vi "VMI_find_peaks.vi"(2 "Acquire Time":i32, 3 "Acquire Queue In":T2, 4 "Peak Find Settings":T1, 6 "Image Queue in":T2, 7 "Peak Position Queue in":T2) -> (0 "error out":errorcluster, 1 "x-y":u32)   [LabVIEW 2020]
uses:
  <vilib>/vision/Image Controls.llb/IMAQ Image.ctl
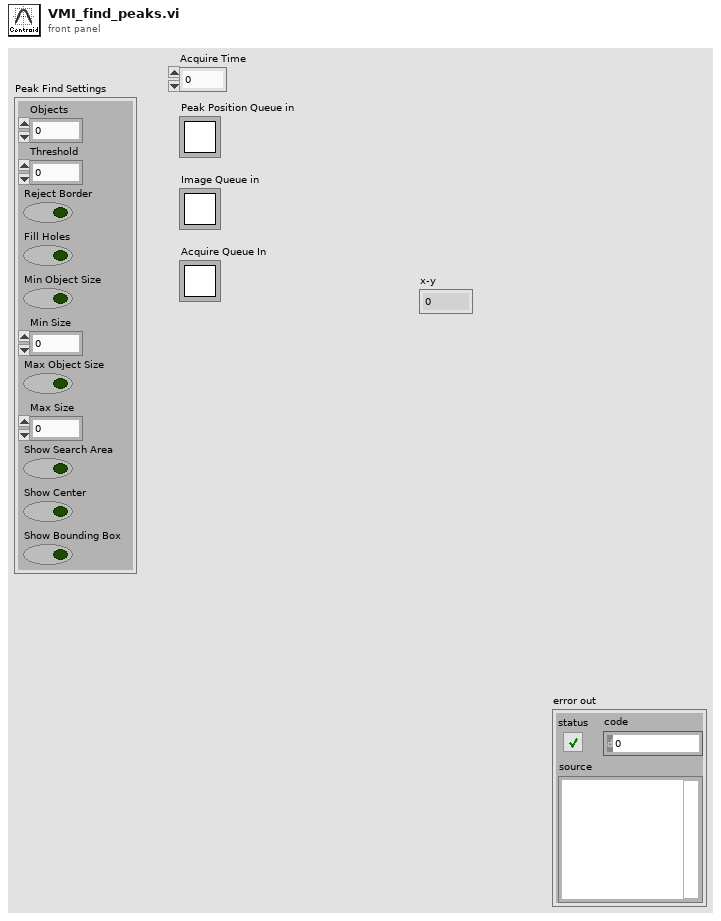
[diagram p1: front panel]
types:
  T1 = cluster{"Objects":u16, "Threshold":i32, "Reject Border":bool, "Fill Holes":bool, "Min Object Size":bool, "Min Size":i32, "Max Object Size":bool, "Max Size":i32, "Show Search Area":bool, "Show Center":bool, "Show Bounding Box":bool}
  T2 = typedef "Queue RefNum" = refnum<k1>
  T3 = typedef "IMAQ Image.ctl" = refnum<image>
  T4 = cluster{"Object Center":cluster{"X":sgl, "Y":sgl}, "Bounding Box":cluster{"X Left":i32, "Y Top":i32, "X Right":i32, "Y Bottom":i32}, "Area":sgl, "Orientation":sgl, "Aspect Ratio":sgl, "Nb Holes":i32}[]
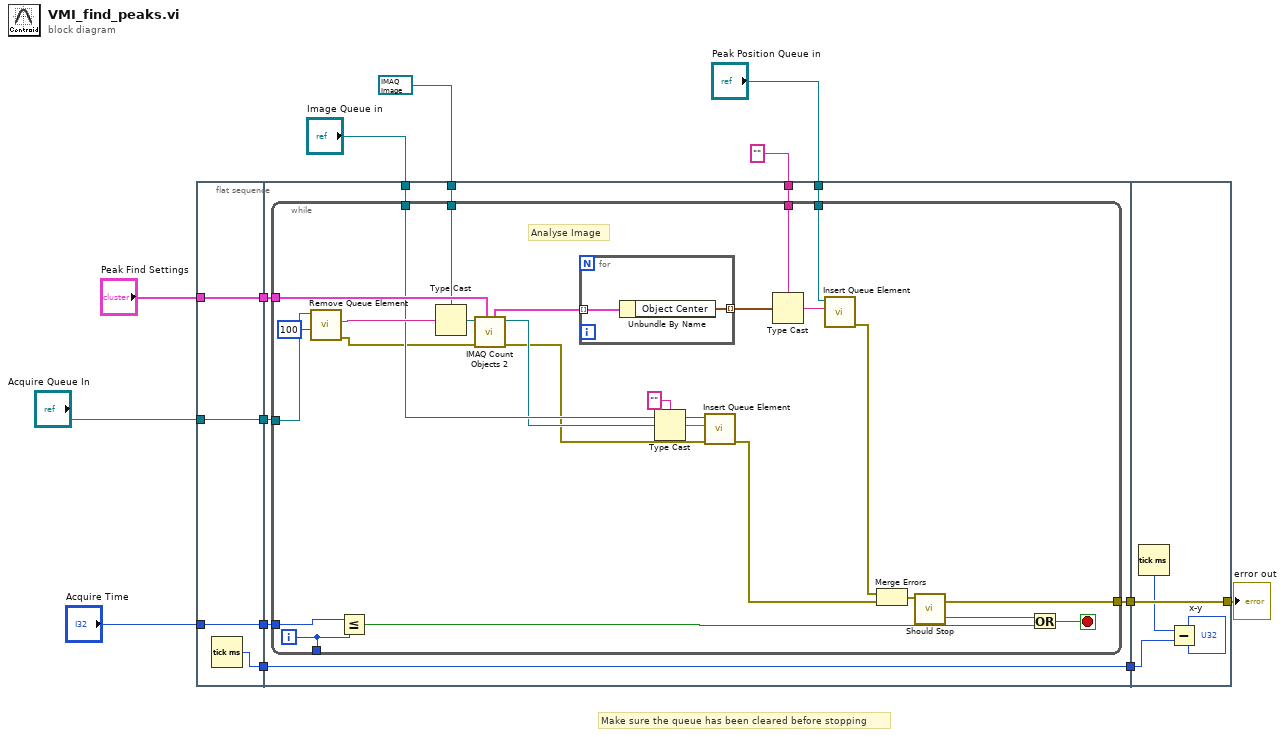
[diagram p0: block diagram]
diagram:
  # "Make sure the queue has been cleared before stopping"
  n1 = flat-sequence {
    tunnel: "Acquire Time" -> [w16]
    tunnel: "Peak Find Settings" -> [w17]
    tunnel: "Acquire Queue In" -> [w18]
    tunnel: [w18] -> w7
    tunnel: [w17] -> w6
    tunnel: [w16] -> w5
    tunnel: [w15] -> w3
    tunnel: "Image Queue in" -> [w27]
    tunnel: "Peak Position Queue in" -> [w23]
    tunnel: [w25] -> w8
    tunnel: w7 -> [w26]
    tunnel: w6 -> [w24]
    tunnel: w5 -> [w22]
    tunnel: [w21] -> w4
    tunnel: w3 -> [w21]
    tunnel: T3 refnum ("Image Out") -> [w20]
    tunnel: "" -> [w19]
    tunnel: [w59] -> w12
    tunnel: w8 -> [w59]
    tunnel: w4 -> [w57]
    frame #0 {
      n2 = Tick Count (ms)() -> (millisecond timer value=w15:u32)
    }
    frame #1 {
      n3 = while {
        tunnel: w26 -> [w40]
        tunnel: w24 -> [w51]
        tunnel: w23 -> [w48]
        tunnel: w27 -> [w46]
        tunnel: [w34] -> w25
        tunnel: w22 -> [w37]
        tunnel: [w33] -> _
        tunnel: w20 -> [w30]
        tunnel: w19 -> [w29]
        i -> [w33]
        stop <- w38 stop-if-true
        # "Analyse Image"
        n4 = call <vilib>:"Remove Queue Element.vi"("ms timeout (-1)"=100, "queue"=w40) -> ("error out"=w44:errorcluster, "queue element"=w53:string)  [unwired: 4 in, 2 out]
        n5 = Less Or Equal?(x=w37, y=w33) -> (x <= y?=w35:bool)
        n6 = Type Cast(type=w30, x=w53) -> (*(type *) &x=w52:T3)
        n7 = call "IMAQ Count Objects 2"("Settings"=w51, "error in (no error)"=w44, "Image"=w52) -> ("error out"=w43:errorcluster, "Image Out"=w45:T3, "Objects"=w50:T4)  [unwired: 4 in, 2 out]
        n8 = for {
          tunnel: w50 -> [w55] mode=indexing
          tunnel: [w54] -> w47 mode=indexing
          n9 = Unbundle By Name(w55) -> ("Object Center"=w54:cluster{"X":sgl, "Y":sgl})
        }
        n10 = Type Cast(type="", x=w45) -> (*(type *) &x=w32:string)
        n11 = call <vilib>:"Insert Queue Element.vi"("error in (no error)"=w43, "queue element"=w32, "queue"=w46) -> ("error out"=w41:errorcluster)  [unwired: 4 in, 2 out]
        n12 = Type Cast(type=w29, x=w47) -> (*(type *) &x=w49:string)
        n13 = call <vilib>:"Insert Queue Element.vi"("queue element"=w49, "queue"=w48) -> ("error out"=w39:errorcluster)  [unwired: 5 in, 2 out]
        n14 = Merge Errors(w39, w41) -> (w42:errorcluster)
        n15 = call "Should Stop.vi"("error in 1"=w42) -> ("error out"=w34:errorcluster, "Stop"=w36:bool)  [unwired: 4 in]
        n16 = Or(x=w36, y=w35) -> (x .or. y?=w38:bool)
      }
    }
    frame #2 {
      n17 = Tick Count (ms)() -> (millisecond timer value=w58:u32)
      n18 = Subtract(x=w58, y=w57) -> (x-y=→"x-y":u32)
    }
  }
  "error out" <- w12
